vi "Thresholds.vi"() -> ()   [LabVIEW 2019, in "Calibration Lib.lvlib"]
uses:
  Calibration Lib.lvlib
  database.lvlib
panel:
  in  "Cancel":bool
  in  "OK":bool
  out "init value":T1(array[cluster])
  in  "Error in 2":errorcluster
  in  "Error in":errorcluster
  out "Name":string
  in  "Grading Threshold":T2(array[cluster])=[{"Disc Number"="Disc 26", "<6.3 mm"=0.0, "6.3-8 mm"=0.0, "8-10 mm"=0.0, "10-12.5 mm"=0.0, "12.5-14 mm"=0.0, "14-16 mm"=0.0, "16-18 mm"=0.0, "18 mm<"=0.0}, {"Disc Number"="Disc 27", "<6.3 mm"=0.0, "6.3-8 mm"=0.0, "8-10 mm"=0.0, "10-12.5 mm"=0.0, "12.5-14 mm"=0.0, "14-16 mm"=0.0, "16-18 mm"=0.0, "18 mm<"=0.0}, {"Disc Number"="Disc 28", "<6.3 mm"=0.0, "6.3-8 mm"=0.0, "8-10 mm"=0.0, "10-12.5 mm"=0.0, "12.5-14 mm"=0.0, "14-16 mm"=0.0, "16-18 mm"=0.0, "18 mm<"=0.0}, {"Disc Number"="Disc 29", "<6.3 mm"=0.0, "6.3-8 mm"=0.0, "8-10 mm"=0.0, "10-12.5 mm"=0.0, "12.5-14 mm"=0.0, "14-16 mm"=0.0, "16-18 mm"=0.0, "18 mm<"=0.0}, {"Disc Number"="Disc 30", "<6.3 mm"=0.0, "6.3-8 mm"=0.0, "8-10 mm"=0.0, "10-12.5 mm"=0.0, "12.5-14 mm"=0.0, "14-16 mm"=0.0, "16-18 mm"=0.0, "18 mm<"=0.0}]
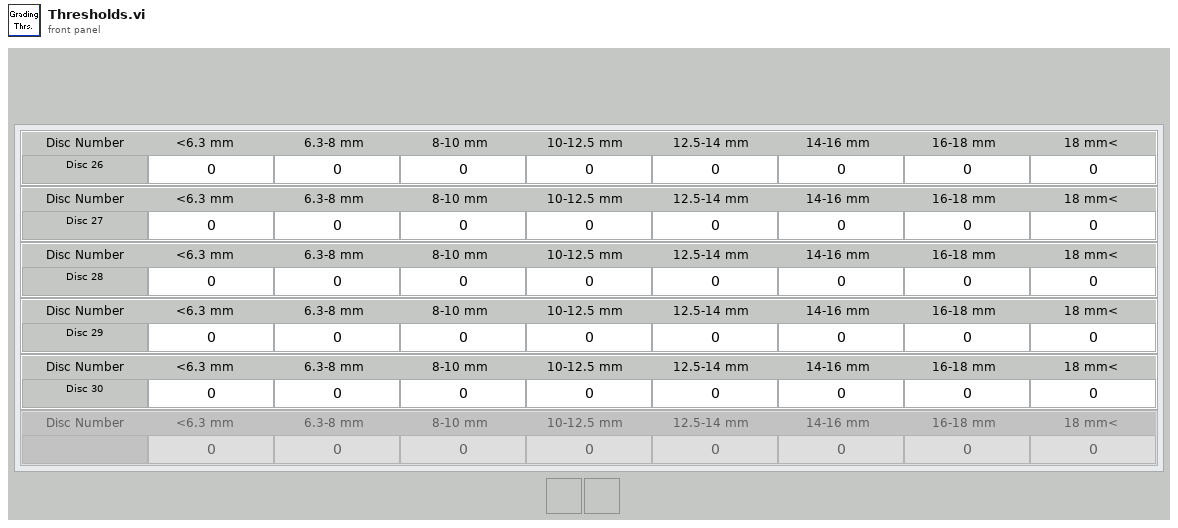
[diagram p1: front panel]
types:
  T1 = cluster{"Disc Number":string, "<6.3 mm":dbl, "6.3-8 mm":dbl, "8-10 mm":dbl, "10-12.5 mm":dbl, "12.5-14 mm":dbl, "14-16 mm":dbl, "16-18 mm":dbl, "<18 mm":dbl}[]
  T2 = cluster{"Disc Number":string, "<6.3 mm":dbl, "6.3-8 mm":dbl, "8-10 mm":dbl, "10-12.5 mm":dbl, "12.5-14 mm":dbl, "14-16 mm":dbl, "16-18 mm":dbl, "18 mm<":dbl}[]
  T3 = cluster{"Disc Number":string, "<6.3 mm":dbl, "6.3-8 mm":dbl, "8-10 mm":dbl, "10-12.5 mm":dbl, "12.5-14 mm":dbl, "14-16 mm":dbl, "16-18 mm":dbl, "<18 mm":dbl}
  T4 = cluster{"Disc Number":string, "<6.3 mm":dbl, "6.3-8 mm":dbl, "8-10 mm":dbl, "10-12.5 mm":dbl, "12.5-14 mm":dbl, "14-16 mm":dbl, "16-18 mm":dbl, "18 mm<":dbl}
  T5 = cluster{"date/time string":string, "date/time string":string, "spreadsheet string":string, "spreadsheet string":string, "spreadsheet string":string, "spreadsheet string":string, "spreadsheet string":string, "spreadsheet string":string}
  T6 = cluster{i32, "date/time string":string, "date/time string":string, "string":string}
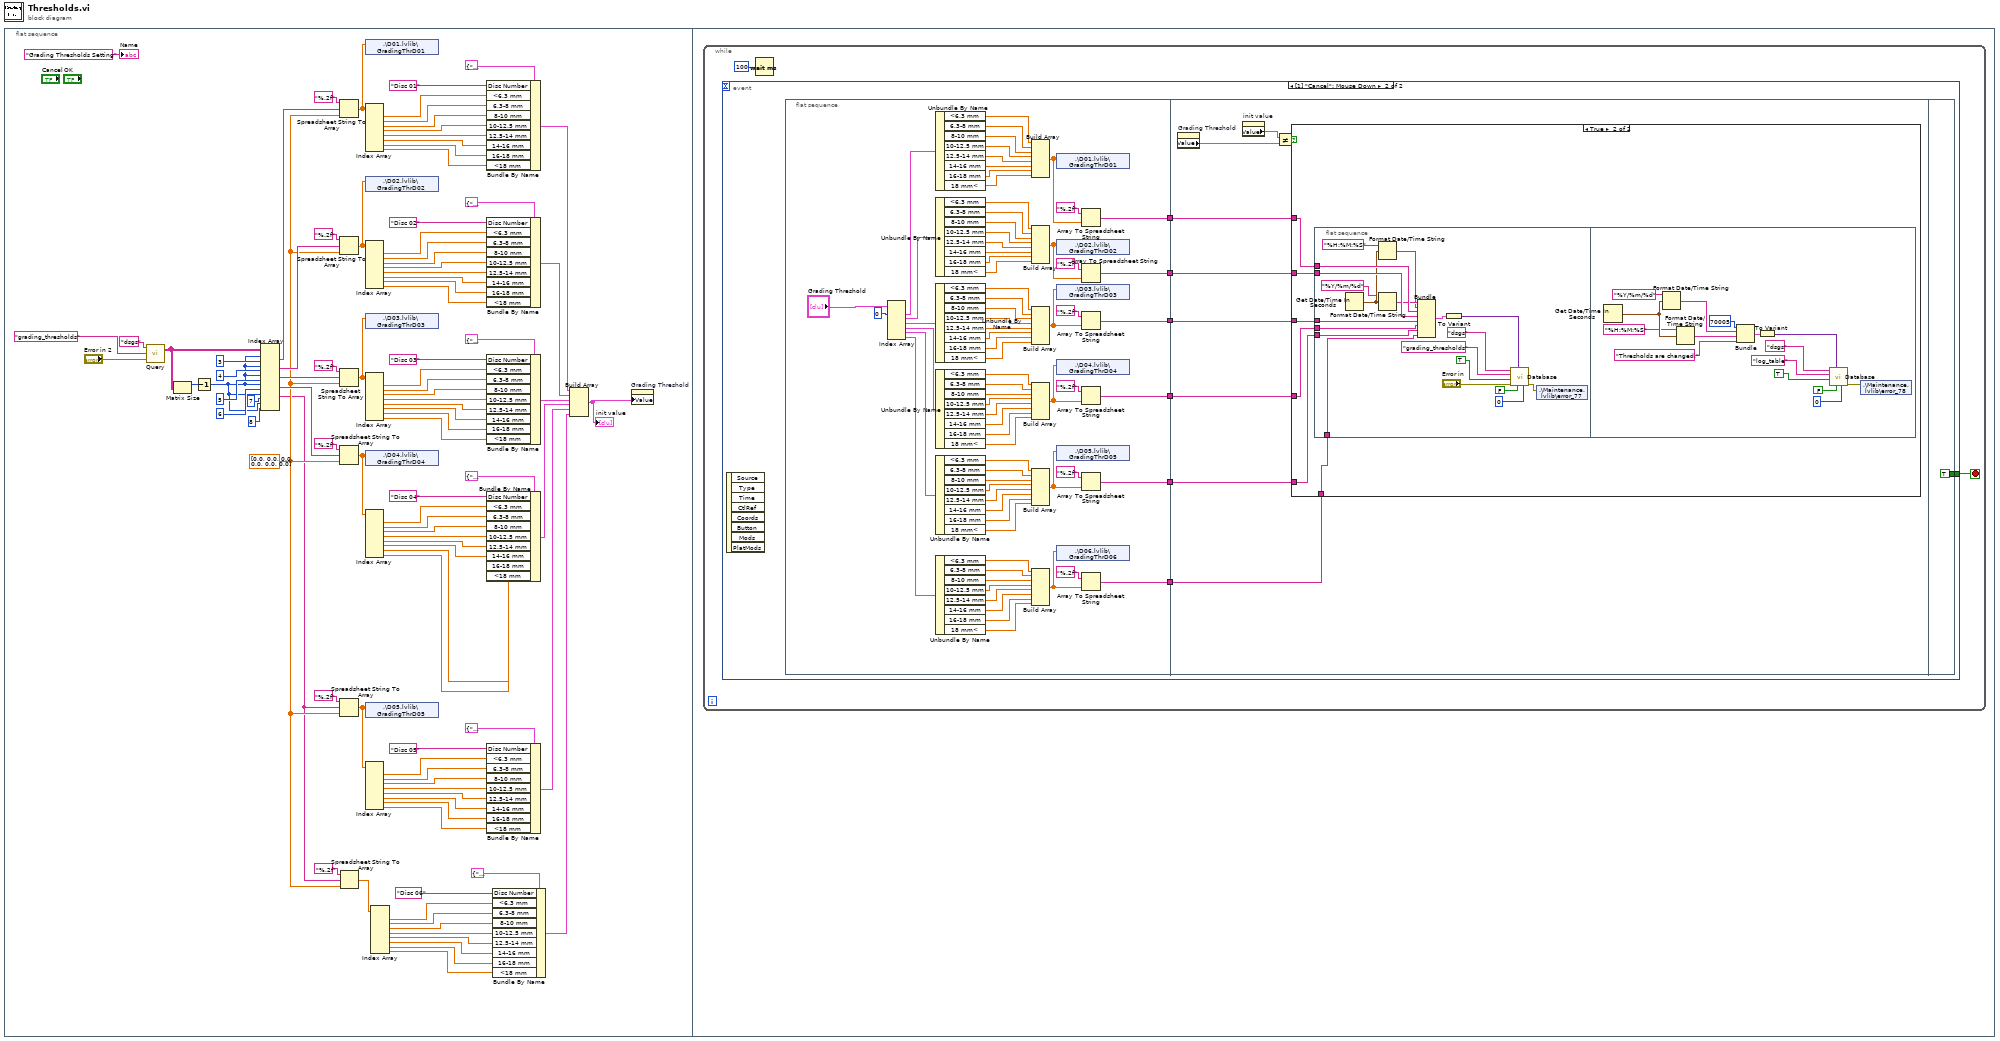
[diagram p0: block diagram]
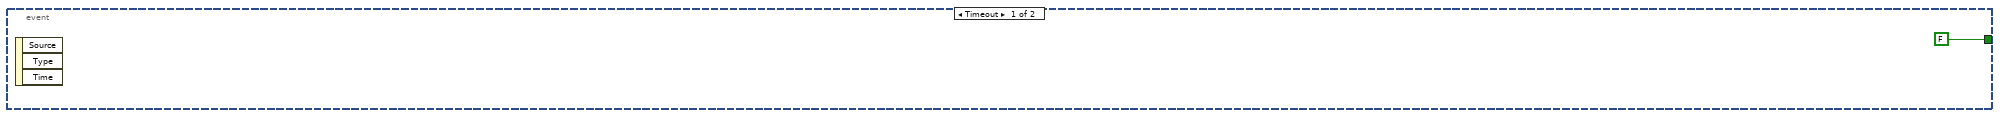
[diagram p2: hidden frame]
diagram:
  n1 = flat-sequence {
    frame #0 {
      w5 = dbl[] [0.0, 0.0, 0.0, 0.0, 0.0, 0.0]
      n2 = call "Query.vi"("Error in"="Error in 2", "Table Name"="grading_thresholds", "Connection Name"="dsgs") -> ("data"=w95:string[][])  [unwired: 1 in, 1 out]
      n3 = Matrix Size(0:w95) -> (1:w94:i32)  [unwired: 1 out]
      n4 = Decrement(x=w94) -> (x-1=w8:i32)
      n5 = Index Array(array=w95, index (row) #1=w8, index (col) #1=3 ("disabled index (col)"), index (row) #2=w8, index (col) #2=4 ("disabled index (col)"), index (row) #3=w8, index (col) #3=5 ("disabled index (col)"), index (row) #4=w8, index (col) #4=6 ("disabled index (col)"), index (row) #5=w8, index (col) #5=7 ("disabled index (col)"), index (row) #6=w8, index (col) #6=8 ("disabled index (col)")) -> (element #1=w88:string, element #2=w82:string, element #3=w81:string, element #4=w80:string, element #5=w4:string)  [unwired: 1 out]
      n6 = Spreadsheet String To Array(format string="%.2f", spreadsheet string=w88, array type (2D Dbl)=w5) -> (array=w22:dbl[])  [unwired: 1 in]
      n7 = Spreadsheet String To Array(format string="%.2f", spreadsheet string=w82, array type (2D Dbl)=w5) -> (array=w21:dbl[])  [unwired: 1 in]
      n8 = Spreadsheet String To Array(format string="%.2f", spreadsheet string=w81, array type (2D Dbl)=w5) -> (array=w20:dbl[])  [unwired: 1 in]
      n9 = Spreadsheet String To Array(format string="%.2f", spreadsheet string=w80, array type (2D Dbl)=w5) -> (array=w19:dbl[])  [unwired: 1 in]
      n10 = Spreadsheet String To Array(format string="%.2f", spreadsheet string=w4, array type (2D Dbl)=w5) -> (array=w18:dbl[])  [unwired: 1 in]
      n11 = Spreadsheet String To Array(format string="%.2f", spreadsheet string=w4, array type (2D Dbl)=w5) -> (array=w3:dbl[])  [unwired: 1 in]
      n12 = shared-variable ".\\D01.lvlib\\GradingThrD01"(w22) -> ()  [unwired: 1 in, 1 out]
      n13 = Index Array(array=w22) -> (element #1=w79:dbl, element #2=w78:dbl, element #3=w77:dbl, element #4=w76:dbl, element #5=w75:dbl, element #6=w74:dbl, element #7=w73:dbl, element #8=w72:dbl)  [unwired: 8 in]
      n14 = shared-variable ".\\D02.lvlib\\GradingThrD02"(w21) -> ()  [unwired: 1 in, 1 out]
      n15 = Index Array(array=w21) -> (element #1=w60:dbl, element #2=w61:dbl, element #3=w62:dbl, element #4=w63:dbl, element #5=w64:dbl, element #6=w65:dbl, element #7=w66:dbl, element #8=w67:dbl)  [unwired: 8 in]
      n16 = shared-variable ".\\D03.lvlib\\GradingThrD03"(w20) -> ()  [unwired: 1 in, 1 out]
      n17 = Index Array(array=w20) -> (element #1=w59:dbl, element #2=w58:dbl, element #3=w57:dbl, element #4=w56:dbl, element #5=w55:dbl, element #6=w54:dbl, element #7=w53:dbl, element #8=w52:dbl)  [unwired: 8 in]
      n18 = shared-variable ".\\D04.lvlib\\GradingThrD04"(w19) -> ()  [unwired: 1 in, 1 out]
      n19 = Index Array(array=w19) -> (element #1=w41:dbl, element #2=w42:dbl, element #3=w43:dbl, element #4=w44:dbl, element #5=w45:dbl, element #6=w46:dbl, element #7=w47:dbl, element #8=w48:dbl)  [unwired: 8 in]
      n20 = shared-variable ".\\D05.lvlib\\GradingThrD05"(w18) -> ()  [unwired: 1 in, 1 out]
      n21 = Index Array(array=w18) -> (element #1=w38:dbl, element #2=w37:dbl, element #3=w36:dbl, element #4=w35:dbl, element #5=w34:dbl, element #6=w33:dbl, element #7=w32:dbl, element #8=w31:dbl)  [unwired: 8 in]
      n22 = Index Array(array=w3) -> (element #1=w9:dbl, element #2=w10:dbl, element #3=w11:dbl, element #4=w12:dbl, element #5=w13:dbl, element #6=w14:dbl, element #7=w15:dbl, element #8=w16:dbl)  [unwired: 8 in]
      n23 = Bundle By Name(cluster=T3 {"Disc Number"="", "<6.3 mm"=0.0, "6.3-8 mm"=0.0, "8-10 mm"=0.0, "10-12.5 mm"=0.0, "12.5-14 mm"=0.0, "14-16 mm"=0.0, "16-18 mm"=0.0, "<18 mm"=0.0}, "Disc Number"="Disc 01" ("format string"), "<6.3 mm"=w79, "6.3-8 mm"=w78, "8-10 mm"=w77, "10-12.5 mm"=w76, "12.5-14 mm"=w75, "14-16 mm"=w74, "16-18 mm"=w73, "<18 mm"=w72) -> (w28:T3)
      n24 = Bundle By Name(cluster=T3 {"Disc Number"="", "<6.3 mm"=0.0, "6.3-8 mm"=0.0, "8-10 mm"=0.0, "10-12.5 mm"=0.0, "12.5-14 mm"=0.0, "14-16 mm"=0.0, "16-18 mm"=0.0, "<18 mm"=0.0}, "Disc Number"="Disc 02" ("format string"), "<6.3 mm"=w60, "6.3-8 mm"=w61, "8-10 mm"=w62, "10-12.5 mm"=w63, "12.5-14 mm"=w64, "14-16 mm"=w65, "16-18 mm"=w66, "<18 mm"=w67) -> (w27:T3)
      n25 = Bundle By Name(cluster=T3 {"Disc Number"="", "<6.3 mm"=0.0, "6.3-8 mm"=0.0, "8-10 mm"=0.0, "10-12.5 mm"=0.0, "12.5-14 mm"=0.0, "14-16 mm"=0.0, "16-18 mm"=0.0, "<18 mm"=0.0}, "Disc Number"="Disc 03" ("format string"), "<6.3 mm"=w59, "6.3-8 mm"=w58, "8-10 mm"=w57, "10-12.5 mm"=w56, "12.5-14 mm"=w55, "14-16 mm"=w54, "16-18 mm"=w53, "<18 mm"=w52) -> (w26:T3)
      n26 = Bundle By Name(cluster=T3 {"Disc Number"="", "<6.3 mm"=0.0, "6.3-8 mm"=0.0, "8-10 mm"=0.0, "10-12.5 mm"=0.0, "12.5-14 mm"=0.0, "14-16 mm"=0.0, "16-18 mm"=0.0, "<18 mm"=0.0}, "Disc Number"="Disc 04" ("format string"), "<6.3 mm"=w41, "6.3-8 mm"=w42, "8-10 mm"=w43, "10-12.5 mm"=w44, "12.5-14 mm"=w45, "14-16 mm"=w46, "16-18 mm"=w47, "<18 mm"=w48) -> (w25:T3)
      n27 = Bundle By Name(cluster=T3 {"Disc Number"="", "<6.3 mm"=0.0, "6.3-8 mm"=0.0, "8-10 mm"=0.0, "10-12.5 mm"=0.0, "12.5-14 mm"=0.0, "14-16 mm"=0.0, "16-18 mm"=0.0, "<18 mm"=0.0}, "Disc Number"="Disc 05" ("format string"), "<6.3 mm"=w38, "6.3-8 mm"=w37, "8-10 mm"=w36, "10-12.5 mm"=w35, "12.5-14 mm"=w34, "14-16 mm"=w33, "16-18 mm"=w32, "<18 mm"=w31) -> (w24:T3)
      n28 = Bundle By Name(cluster=T3 {"Disc Number"="", "<6.3 mm"=0.0, "6.3-8 mm"=0.0, "8-10 mm"=0.0, "10-12.5 mm"=0.0, "12.5-14 mm"=0.0, "14-16 mm"=0.0, "16-18 mm"=0.0, "<18 mm"=0.0}, "Disc Number"="Disc 06" ("format string"), "<6.3 mm"=w9, "6.3-8 mm"=w10, "8-10 mm"=w11, "10-12.5 mm"=w12, "12.5-14 mm"=w13, "14-16 mm"=w14, "16-18 mm"=w15, "<18 mm"=w16) -> (w1:T3)
      n29 = Build Array(w28, w27, w26, w25, w24, w1) -> (w23:T1)
      "init value" <- w23
      n30 = property on="Grading Threshold" class="Arr (strict)"("Value"=w23) -> ()  [unwired: 2 in, 2 out]
      "Name" <- "Grading Thresholds Setting" ("Name")
    }
    frame #1 {
      n31 = while {
        stop <- w100 stop-if-true
        n32 = event shown="[1] \"Cancel\": Mouse Down" {
          selector: _ -> [_ _]
          dyn-events: _ -> [_ _]
          timeout: _ -> [_ _]
          tunnel: [FALSE w108] -> w100
          event Timeout {
            n33 = event-data() -> ()  [unwired: 1 in, 3 out]
          }
          event "Cancel": Mouse Down {
            n34 = event-data() -> ()  [unwired: 1 in, 8 out]
            n35 = flat-sequence {
              tunnel: [w125] -> w107
              tunnel: [w124] -> w106
              tunnel: [w123] -> w105
              tunnel: [w122] -> w104
              tunnel: [w121] -> w103
              tunnel: [w109] -> w102
              tunnel: w107 -> [w191]
              tunnel: w106 -> [w190]
              tunnel: w105 -> [w189]
              tunnel: w104 -> [w188]
              tunnel: w103 -> [w187]
              tunnel: w102 -> [w183]
              tunnel: [TRUE] -> w108
              frame #0 {
                n36 = Index Array(array="Grading Threshold", index #1=0 ("index")) -> (element #1=w133:T4, element #2=w134:T4, element #3=w135:T4, element #4=w136:T4, element #5=w137:T4, element #6=w110:T4)  [unwired: 5 in]
                n37 = Unbundle By Name(w133) -> ("<6.3 mm"=w138:dbl, "6.3-8 mm"=w139:dbl, "8-10 mm"=w140:dbl, "10-12.5 mm"=w141:dbl, "12.5-14 mm"=w142:dbl, "14-16 mm"=w143:dbl, "16-18 mm"=w144:dbl, "18 mm<"=w145:dbl)
                n38 = Unbundle By Name(w134) -> ("<6.3 mm"=w146:dbl, "6.3-8 mm"=w147:dbl, "8-10 mm"=w153:dbl, "10-12.5 mm"=w152:dbl, "12.5-14 mm"=w151:dbl, "14-16 mm"=w150:dbl, "16-18 mm"=w149:dbl, "18 mm<"=w148:dbl)
                n39 = Unbundle By Name(w135) -> ("<6.3 mm"=w154:dbl, "6.3-8 mm"=w161:dbl, "8-10 mm"=w160:dbl, "10-12.5 mm"=w159:dbl, "12.5-14 mm"=w158:dbl, "14-16 mm"=w157:dbl, "16-18 mm"=w156:dbl, "18 mm<"=w155:dbl)
                n40 = Unbundle By Name(w136) -> ("<6.3 mm"=w163:dbl, "6.3-8 mm"=w164:dbl, "8-10 mm"=w165:dbl, "10-12.5 mm"=w166:dbl, "12.5-14 mm"=w167:dbl, "14-16 mm"=w168:dbl, "16-18 mm"=w169:dbl, "18 mm<"=w162:dbl)
                n41 = Unbundle By Name(w137) -> ("<6.3 mm"=w170:dbl, "6.3-8 mm"=w177:dbl, "8-10 mm"=w176:dbl, "10-12.5 mm"=w175:dbl, "12.5-14 mm"=w174:dbl, "14-16 mm"=w173:dbl, "16-18 mm"=w172:dbl, "18 mm<"=w171:dbl)
                n42 = Unbundle By Name(w110) -> ("<6.3 mm"=w119:dbl, "6.3-8 mm"=w112:dbl, "8-10 mm"=w113:dbl, "10-12.5 mm"=w114:dbl, "12.5-14 mm"=w115:dbl, "14-16 mm"=w116:dbl, "16-18 mm"=w117:dbl, "18 mm<"=w118:dbl)
                n43 = Build Array(w138, w139, w140, w141, w142, w143, w144, w145) -> (w178:dbl[])
                n44 = Build Array(w146, w147, w153, w152, w151, w150, w149, w148) -> (w179:dbl[])
                n45 = Build Array(w154, w161, w160, w159, w158, w157, w156, w155) -> (w180:dbl[])
                n46 = Build Array(w163, w164, w165, w166, w167, w168, w169, w162) -> (w181:dbl[])
                n47 = Build Array(w170, w177, w176, w175, w174, w173, w172, w171) -> (w182:dbl[])
                n48 = Build Array(w119, w112, w113, w114, w115, w116, w117, w118) -> (w111:dbl[])
                n49 = shared-variable ".\\D01.lvlib\\GradingThrD01"(w178) -> ()  [unwired: 1 in, 1 out]
                n50 = shared-variable ".\\D02.lvlib\\GradingThrD02"(w179) -> ()  [unwired: 1 in, 1 out]
                n51 = shared-variable ".\\D03.lvlib\\GradingThrD03"(w180) -> ()  [unwired: 1 in, 1 out]
                n52 = shared-variable ".\\D04.lvlib\\GradingThrD04"(w181) -> ()  [unwired: 1 in, 1 out]
                n53 = shared-variable ".\\D05.lvlib\\GradingThrD05"(w182) -> ()  [unwired: 1 in, 1 out]
                n54 = shared-variable ".\\D06.lvlib\\GradingThrD06"(w111) -> ()  [unwired: 1 in, 1 out]
                n55 = Array To Spreadsheet String(array=w178, 3:"%.2f" ("format string")) -> (spreadsheet string=w125:string)  [unwired: 1 in]
                n56 = Array To Spreadsheet String(array=w179, 3:"%.2f" ("format string")) -> (spreadsheet string=w124:string)  [unwired: 1 in]
                n57 = Array To Spreadsheet String(array=w180, 3:"%.2f" ("format string")) -> (spreadsheet string=w123:string)  [unwired: 1 in]
                n58 = Array To Spreadsheet String(array=w181, 3:"%.2f" ("format string")) -> (spreadsheet string=w122:string)  [unwired: 1 in]
                n59 = Array To Spreadsheet String(array=w182, 3:"%.2f" ("format string")) -> (spreadsheet string=w121:string)  [unwired: 1 in]
                n60 = Array To Spreadsheet String(array=w111, 3:"%.2f" ("format string")) -> (spreadsheet string=w109:string)  [unwired: 1 in]
              }
              frame #1 {
                n61 = property on="Grading Threshold" class="Arr (strict)"() -> ("Value"=w185:T2)  [unwired: 2 in, 2 out]
                n62 = property on="init value" class="Arr (strict)"() -> ("Value"=w186:T1)  [unwired: 2 in, 2 out]
                n63 = Not Equal?(x=w186, y=w185) -> (x != y?=w184:bool)
                n64 = case shown="True" w184 {
                  tunnel: w191 -> [_ w197]
                  tunnel: w190 -> [_ w196]
                  tunnel: w189 -> [_ w195]
                  tunnel: w188 -> [_ w194]
                  tunnel: w187 -> [_ w193]
                  tunnel: w183 -> [_ w192]
                  frame False {
                  }
                  frame True {
                    n65 = flat-sequence {
                      tunnel: w197 -> [w211]
                      tunnel: w196 -> [w210]
                      tunnel: w195 -> [w209]
                      tunnel: w194 -> [w208]
                      tunnel: w193 -> [w207]
                      tunnel: w192 -> [w198]
                      frame #0 {
                        n66 = Get Date/Time In Seconds() -> (seconds since 1Jan1904=w206:timestamp)
                        n67 = Format Date/Time String(time format string (%c)="%H:%M:%S", seconds (now)=w206) -> (date/time string=w202:string)  [unwired: 1 in]
                        n68 = Format Date/Time String(time format string (%c)="%Y/%m/%d", seconds (now)=w206) -> (date/time string=w203:string)  [unwired: 1 in]
                        n69 = Bundle("date/time string"=w203, "date/time string"=w202, "spreadsheet string"=w211, "spreadsheet string"=w210, "spreadsheet string"=w209, "spreadsheet string"=w208, "spreadsheet string"=w207, "spreadsheet string"=w198) -> (w201:T5)  [unwired: 1 in]
                        n70 = To Variant(anything=w201) -> (Variant=w200:variant)
                        n71 = call "Database.vi"("Maximum Row"=u64 0 ("Storage Time (Day)"), "Delete row?"=FALSE, "Data"=w200, "Error in"="Error in", "Auto Increment ID?"=TRUE, "Table"="grading_thresholds", "Connection"="dsgs") -> ("Error out"=w199:errorcluster)  [unwired: 4 in]
                        n72 = shared-variable ".\\Maintenance.lvlib\\error_77"(w199) -> ()  [unwired: 1 in, 1 out]
                      }
                      frame #1 {
                        n73 = Get Date/Time In Seconds() -> (seconds since 1Jan1904=w228:timestamp)
                        n74 = Format Date/Time String(time format string (%c)="%Y/%m/%d", seconds (now)=w228) -> (date/time string=w229:string)  [unwired: 1 in]
                        n75 = Format Date/Time String(time format string (%c)="%H:%M:%S", seconds (now)=w228) -> (date/time string=w230:string)  [unwired: 1 in]
                        n76 = Bundle(70005, "date/time string"=w229, "date/time string"=w230, "string"="Thresholds are changed.") -> (w231:T6)  [unwired: 1 in]
                        n77 = To Variant(anything=w231) -> (Variant=w232:variant)
                        n78 = call "Database.vi"("Maximum Row"=u64 0 ("Storage Time (Day)"), "Delete row?"=FALSE, "Data"=w232, "Auto Increment ID?"=TRUE, "Table"="log_table" ("table"), "Connection"="dsgs" ("table")) -> ("Error out"=w218:errorcluster)  [unwired: 5 in]
                        n79 = shared-variable ".\\Maintenance.lvlib\\error_78"(w218) -> ()  [unwired: 1 in, 1 out]
                      }
                    }
                  }
                }
              }
              frame #2 {
              }
            }
          }
        }
        n80 = Wait (ms)(milliseconds to wait=u32 100) -> ()  [unwired: 1 out]
      }
    }
  }
